vi "Change_speed.vi"(1 "ST_SPD":dbl, 2 "MC-BonOMM VRN":refnum<visa-resource-name>) -> (0 "Connected?":bool)   [LabVIEW 2019]
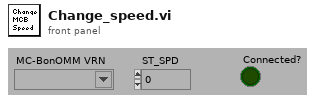
[diagram p1: front panel]
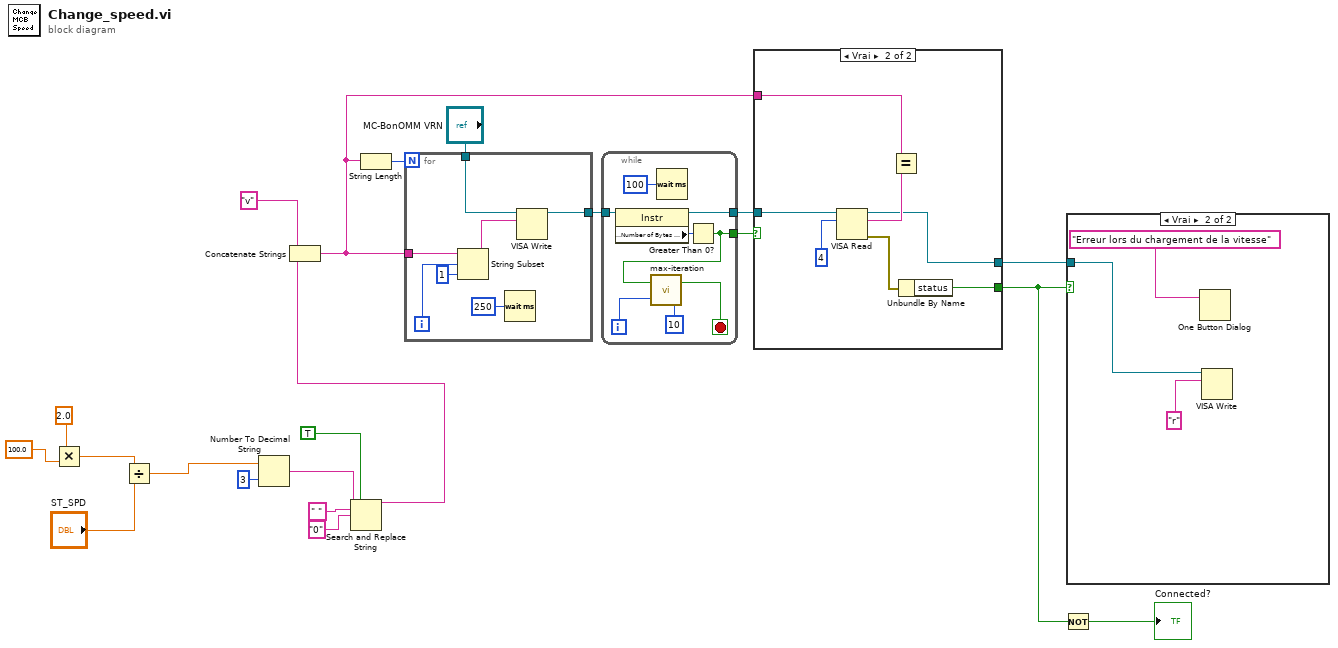
[diagram p0: block diagram]
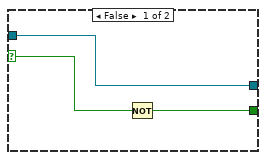
[diagram p3: hidden frame]
diagram:
  n1 = Multiply(x=2.0 ("y"), y=100.0) -> (x*y=w10:dbl)
  n2 = Divide(x=w10, y="ST_SPD") -> (x/y=w12:dbl)
  n3 = Number To Decimal String(number=w12, width (-)=i16 3) -> (decimal integer string=w3:string)
  n4 = Search and Replace String(replace all?=TRUE ("replace all? (F)"), input string=w3, search string=" ", replace string="0" ("replace string (\"\")")) -> (result string=w7:string)  [unwired: 4 in, 3 out]
  n5 = Concatenate Strings("v" ("Commande"), w7) -> (w15:string)
  n6 = String Length(string=w15) -> (length=w14:i32)
  n7 = for {
    N: w14 -> [_]
    tunnel: w15 -> [w26]
    tunnel: "MC-BonOMM VRN" -> [w24]
    tunnel: [w23] -> w16
    i -> [w27]
    n8 = String Subset(string=w26, offset (0)=w27, length (rest)=1 ("length (rest)")) -> (substring=w25:string)
    n9 = Wait (ms)(milliseconds to wait=u32 250) -> ()  [unwired: 1 out]
    n10 = VISA Write(VISA resource name=w24, write buffer=w25) -> (VISA resource name out=w23:refnum<visa-resource-name>)  [unwired: 1 in, 2 out]
  }
  n11 = while {
    tunnel: w16 -> [w36]
    tunnel: [w35] -> w17
    tunnel: [w32] -> w18
    i -> [w33]
    stop <- w31 stop-if-true
    n12 = property class="Instr"(reference=w36) -> (reference out=w35:refnum<visa-resource-name>, "Serial Settings:Number of Bytes at Serial Port"=w34:u32)  [unwired: 1 in, 1 out]
    n13 = Wait (ms)(milliseconds to wait=u32 100) -> ()  [unwired: 1 out]
    n14 = Greater Than 0?(x=w34) -> (x > 0?=w32:bool)
    n15 = call "max-iteration.vi"("i max"=10, "i act"=w33, "Valeur entrante"=w32) -> ("break ?"=w31:bool)
  }
  n16 = case shown="Vrai" w18 {
    selector: w18 -> [w38 _]
    tunnel: w15 -> [_ w43]
    tunnel: w17 -> [w37 w42]
    tunnel: [w39 w41] -> w21
    tunnel: [w37 w40] -> w19
    frame False {
      n17 = Not(x=w38) -> (.not. x?=w39:bool)
    }
    frame True {
      n18 = VISA Read(VISA resource name=w42, byte count=u32 4) -> (VISA resource name out=w40:refnum<visa-resource-name>, read buffer=w44:string, error out=w45:errorcluster)  [unwired: 1 in, 1 out]
      n19 = Equal?(x=w43, y=w44) -> ()  [unwired: 1 out]
      n20 = Unbundle By Name(w45) -> ("status"=w41:bool)
    }
  }
  n21 = Not(x=w21) -> (.not. x?=→"Connected?":bool)
  n22 = case shown="Vrai" w21 {
    tunnel: w19 -> [_ w47]
    frame False {
    }
    frame True {
      n23 = One Button Dialog(message="Erreur lors du chargement de la vitesse") -> ()  [unwired: 1 in, 1 out]
      n24 = VISA Write(VISA resource name=w47, write buffer="r") -> ()  [unwired: 1 in, 3 out]
    }
  }
